vi "ADIS16448 Loop Manage Cal Buffer.vi"(7 "Cmd":T1, 9 "Sample Count":i32, 11 "Data In":dbl[](array[numeric])) -> (3 "Cal Offset Out":dbl[](array[numeric]))   [LabVIEW 2019]
uses:
  Typedef/ADIS16448 Call Buffer Cmd.ctl
  <vilib>/Analysis/baseanly.llb/Mean.vi
  <vilib>/Analysis/baseanly.llb/Mean (DBL).vi
panel:
  # "NON-REENTRANT"
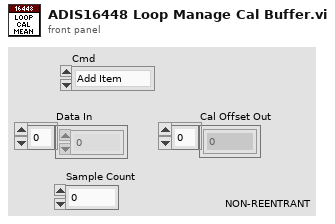
[diagram p1: front panel]
types:
  T1 = typedef "ADIS16448 Call Buffer Cmd.ctl" = enum16{"Add Item ", "Calculate"}
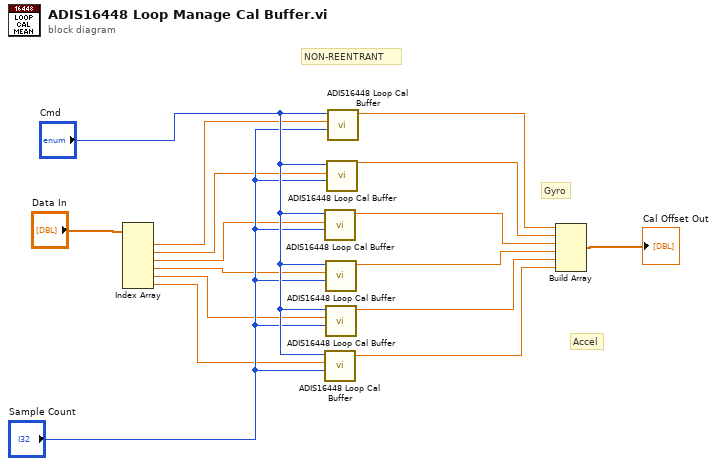
[diagram p0: block diagram]
diagram:
  # "NON-REENTRANT"
  # "Accel"
  # "Gyro"
  n1 = Index Array(array="Data In") -> (element #1=w13:dbl, element #2=w12:dbl, element #3=w11:dbl, element #4=w10:dbl, element #5=w9:dbl, element #6=w8:dbl)  [unwired: 6 in]
  n2 = call "ADIS16448 Loop Cal Buffer.vi"("Max Samples"="Sample Count", "New Value"=w11, "Cmd"="Cmd") -> ("Mean"=w4:dbl)  [unwired: 8 in]
  n3 = call "ADIS16448 Loop Cal Buffer.vi"("Max Samples"="Sample Count", "New Value"=w8, "Cmd"="Cmd") -> ("Mean"=w1:dbl)  [unwired: 8 in]
  n4 = call "ADIS16448 Loop Cal Buffer.vi"("Max Samples"="Sample Count", "New Value"=w10, "Cmd"="Cmd") -> ("Mean"=w3:dbl)  [unwired: 8 in]
  n5 = call "ADIS16448 Loop Cal Buffer.vi"("Max Samples"="Sample Count", "New Value"=w9, "Cmd"="Cmd") -> ("Mean"=w2:dbl)  [unwired: 8 in]
  n6 = call "ADIS16448 Loop Cal Buffer.vi"("Max Samples"="Sample Count", "New Value"=w12, "Cmd"="Cmd") -> ("Mean"=w5:dbl)  [unwired: 8 in]
  n7 = call "ADIS16448 Loop Cal Buffer.vi"("Max Samples"="Sample Count", "New Value"=w13, "Cmd"="Cmd") -> ("Mean"=w6:dbl)  [unwired: 8 in]
  n8 = Build Array(w6, w5, w4, w3, w2, w1) -> (→"Cal Offset Out":dbl[])
